vi "Select_Table_Vaule Enable_Disable.vi"(9 "Action":string, 11 "Table":string[][](array[string])) -> (1 "Enable":bool, 3 "vaule":string[](array[string]))   [LabVIEW 2017]
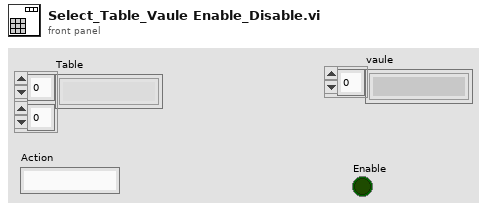
[diagram p1: front panel]
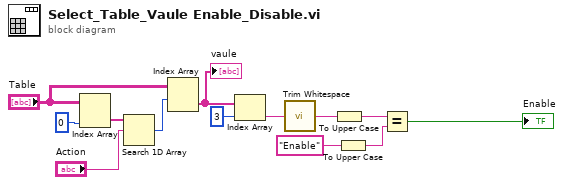
[diagram p0: block diagram]
diagram:
  n1 = Index Array(array="Table", index (col)=0 ("禁用的索引 (列)")) -> (element=w12:string[])  [unwired: 1 in]
  n2 = Search 1D Array(1D array=w12, element="Action") -> (index of element=w9:i32)  [unwired: 1 in]
  n3 = Index Array(array="Table", index (row)=w9) -> (element=w4:string[])  [unwired: 1 in]
  "vaule" <- w4
  n4 = Index Array(array=w4, index=3 ("索引")) -> (element=w5:string)
  n5 = call <vilib>:"Trim Whitespace.vi"("string"=w5) -> ("trimmed string"=w7:string)  [unwired: 1 in]
  n6 = To Upper Case(1:w7) -> (0:w3:string)
  n7 = To Upper Case(1:"Enable" ("y")) -> (0:w2:string)
  n8 = Equal?(x=w3, y=w2) -> (x = y?=→"Enable":bool)
